vi "lvlib to string files.vi"(4 "Export Diagram":bool, 6 "Create Captions":bool=TRUE, 8 "error in (no error)":errorcluster, 10 "Library String Files Root":path=path "E:/VI2String/Test Project/Test Project.lvproj", 11 "lvlib Path":path) -> (0 "error out":errorcluster)   [LabVIEW 2022 SP3]
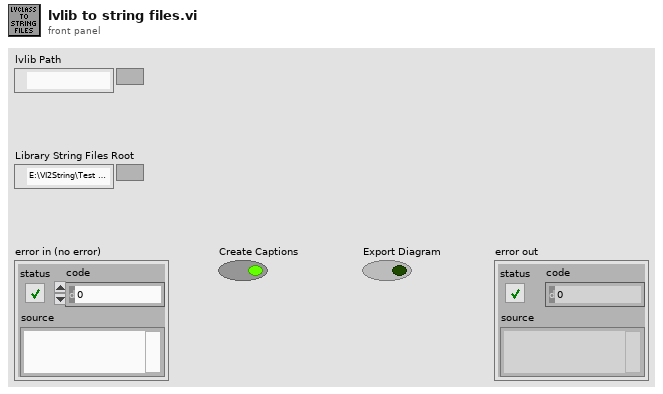
[diagram p1: front panel]
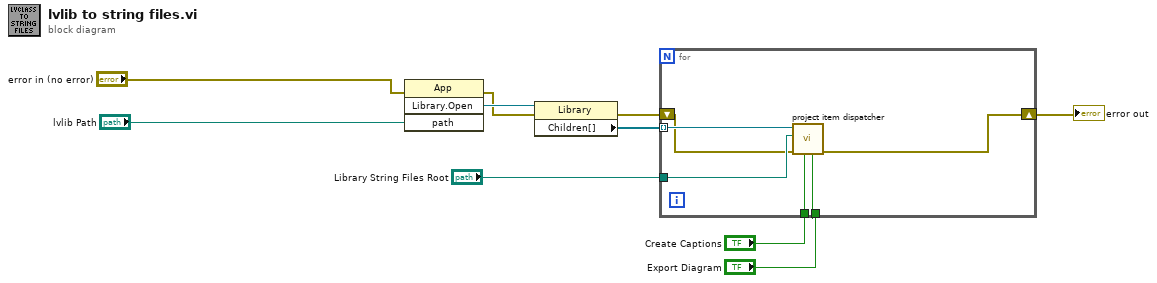
[diagram p0: block diagram]
diagram:
  n1 = invoke class="App" method="Library.Open"(error in="error in (no error)", "path"="lvlib Path") -> (error out=w3:errorcluster, "Open Library"=w9:refnum<vi>)  [unwired: 2 in, 2 out]
  n2 = property class="Library"(reference=w9, error in=w3) -> (error out=w2:errorcluster, "Children[]"=w8:refnum<vi>[])  [unwired: 1 out]
  n3 = for {
    tunnel: w8 -> [w16] mode=indexing
    tunnel: "Create Captions" -> [w15]
    tunnel: "Export Diagram" -> [w14]
    tunnel: "Library String Files Root" -> [w13]
    shift-right: [w11] -> w1
    shift-left: w2 -> [w12]
    n4 = call "project item dispatcher.vi"("Export Diagram"=w14, "Create Captions"=w15, "error in (no error)"=w12, "String Files Root"=w13, "ProjectItem in"=w16) -> ("error out"=w11:errorcluster)  [unwired: 6 in]
  }
  "error out" <- w1
